vi "diagnostics.vi"(0 "Path Data":T1={"Path"=[], "Target Velocities"=[], "Robot Location"=[], "Relative Robot Angle (rad)"=0.0, "Curvature"=0.0, "Lookahead Point"=[3064.399009129367, 18229.833030071386], "Lookahead Index"=8.422809037111724, "Closest Point"=[], "Closest Point Index"=0, "Left Velocity"=0.0, "Right Velocity"=0.0, "Left Encoder Vel"=0, "Right Encoder Vel"=0, "Left Encoder Pos"=0, "Right Encoder Pos"=0, "Inital Robot Angle (deg)"=0.0}) -> (4 "Path":T4(graph)=[{"Smooth Path"=[0.0, 3.9831976339745525, 8.918786774310743, 15.996756278926227, 26.94310215462526, 44.45175679243214, 72.85576199340136, 119.21333672590853, 195.06952147459873, 319.3449114169336, 523.0654465520985, 857.1178508590853, 1404.971654642396, 2303.5684955547395, 3415.918100969553, 4658.468244850319, 5980.216850342943, 7349.961644912561, 8748.499353660785, 10163.825114581763, 11588.130666803412, 13015.85297046767, 14442.283167634836, 15862.389189218296, 17269.55815292861, 18653.942887255045, 20000.0], "Smooth Path"=[0.0, 2604.6593521886216, 5208.4834070465695, 7810.428161388078, 10408.979451847843, 13001.776283234469, 15585.016727668002, 18152.511956181766, 20694.135215630122, 23193.291890529486, 25622.77148689383, 27937.944042539046, 30065.60256829882, 32209.66168633789, 34363.622817575204, 36523.46279208931, 38686.62801955882, 40851.39631476969, 43016.44613594504, 45180.526806154805, 47342.144596973565, 49499.19086028001, 51648.41344856078, 53784.60445996854, 55899.29829439407, 57978.65493411005, 60000.0]}, {"Smooth Path"=[-155.34781165121697, -32.634161371312175], "Smooth Path"=[-10126.308473842537, -2127.2496942088364]}, {"Smooth Path"=[0.0], "Smooth Path"=[0.0]}, {"Smooth Path"=[0.0, -155.34781165121697], "Smooth Path"=[0.0, -10126.308473842537]}], 6 "Robot Angle (deg)":dbl=-0.87890625, 8 "Target Velocities":cluster{dbl, dbl}(graph)={850.0, 850.0}, 10 "Left Velocity":T2(graph)={"Quadrature Velocity"=0, "Left Velocity"=850.0}, 15 "Right Velocity":T3(graph)={"Quadrature Velocity"=0, "Right Velocity"=850.0})   [LabVIEW 2018]
uses:
  path data.ctl
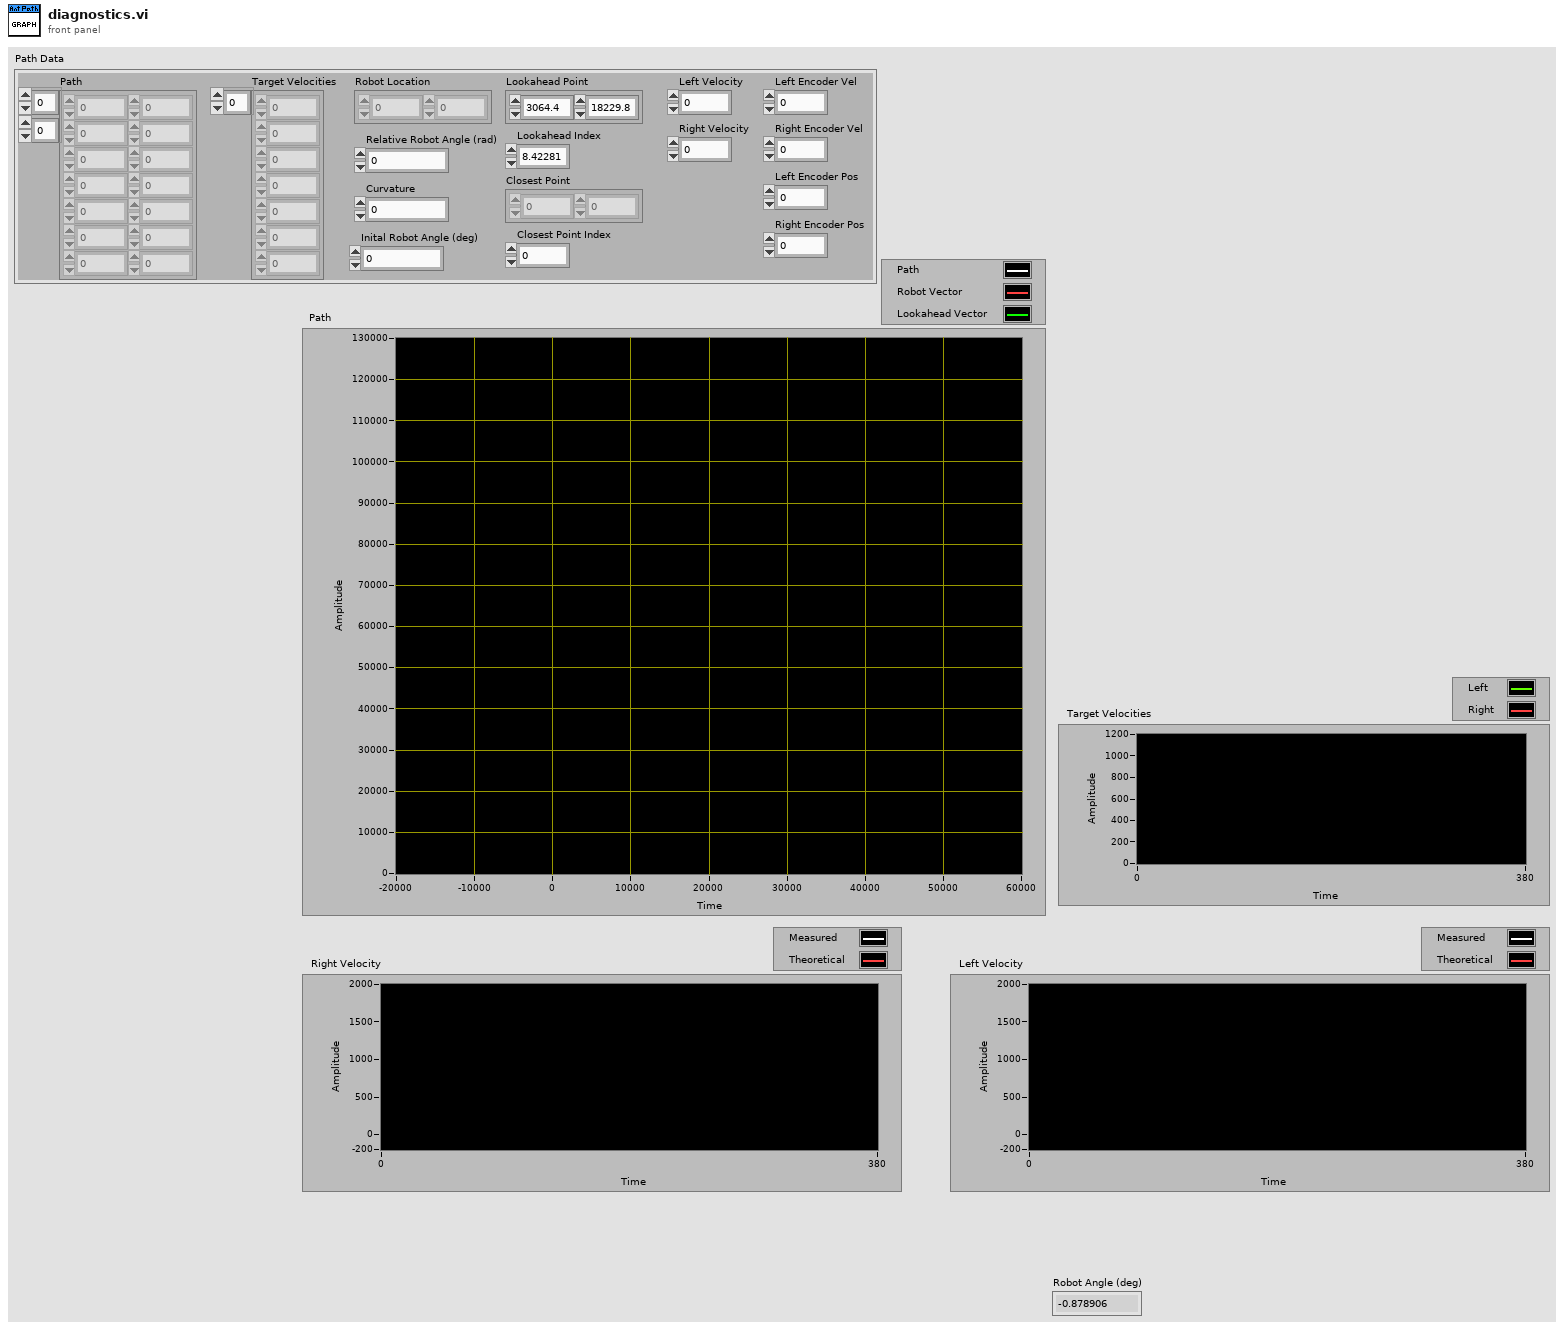
[diagram p1: front panel]
types:
  T1 = typedef "path data.ctl" = cluster{"Path":dbl[][], "Target Velocities":dbl[], "Robot Location":dbl[], "Relative Robot Angle (rad)":dbl, "Curvature":dbl, "Lookahead Point":dbl[], "Lookahead Index":dbl, "Closest Point":dbl[], "Closest Point Index":i32, "Left Velocity":dbl, "Right Velocity":dbl, "Left Encoder Vel":i32, "Right Encoder Vel":i32, "Left Encoder Pos":i32, "Right Encoder Pos":i32, "Inital Robot Angle (deg)":dbl}
  T2 = cluster{"Quadrature Velocity":i32, "Left Velocity":dbl}
  T3 = cluster{"Quadrature Velocity":i32, "Right Velocity":dbl}
  T4 = cluster{"Smooth Path":dbl[], "Smooth Path":dbl[]}[]
  T5 = cluster{"Left Velocity":dbl, "Right Velocity":dbl}
  T6 = cluster{"Left Encoder Vel":i32, "Left Velocity":dbl}
  T7 = cluster{"Right Encoder Vel":i32, "Right Velocity":dbl}
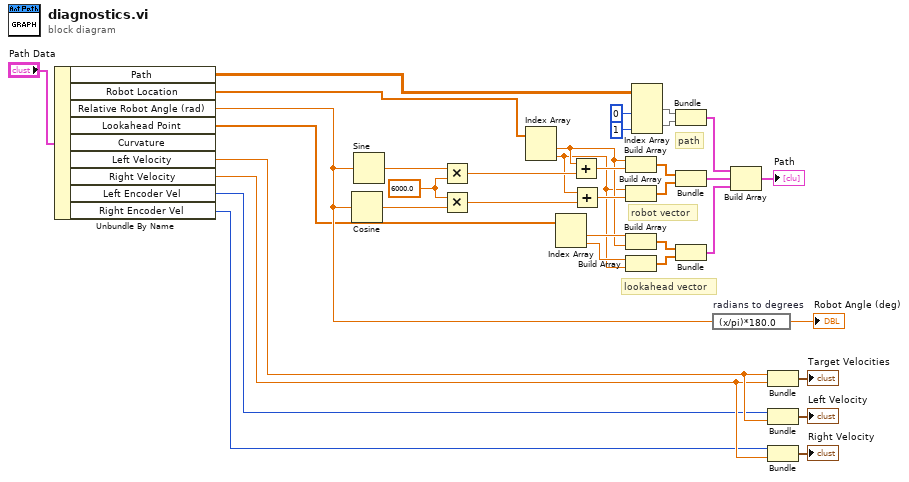
[diagram p0: block diagram]
diagram:
  w27 = 6000.0
  # "lookahead vector"
  # "robot vector"
  # "path"
  n1 = Unbundle By Name("Path Data") -> ("Path"=w8:dbl[][], "Robot Location"=w7:dbl[], "Relative Robot Angle (rad)"=w6:dbl, "Lookahead Point"=w5:dbl[], "Left Velocity"=w4:dbl, "Right Velocity"=w3:dbl, "Left Encoder Vel"=w2:i32, "Right Encoder Vel"=w1:i32)  [unwired: 1 out]
  n2 = Cosine(x=w6) -> (cos(x)=w28:dbl)
  n3 = Sine(x=w6) -> (sin(x)=w29:dbl)
  n4 = Multiply(x=w29, y=w27) -> (x*y=w26:dbl)
  n5 = Multiply(x=w27, y=w28) -> (x*y=w25:dbl)
  n6 = Index Array(array=w7) -> (element #1=w15:dbl, element #2=w14:dbl)  [unwired: 2 in]
  n7 = Index Array(array=w5) -> (element #1=w20:dbl, element #2=w18:dbl)  [unwired: 2 in]
  n8 = Add(x=w15, y=w26) -> (x+y=w24:dbl)
  n9 = Add(x=w14, y=w25) -> (x+y=w23:dbl)
  n10 = Build Array(w15, w24) -> (w33:dbl[])
  n11 = Build Array(w14, w23) -> (w32:dbl[])
  n12 = Build Array(w20, w15) -> (w22:dbl[])
  n13 = Build Array(w18, w14) -> (w21:dbl[])
  n14 = Index Array(array=w8, index (col) #1=0 ("disabled index (col)"), index (col) #2=1 ("index (col)")) -> (element #1=w36:dbl[], element #2=w16:dbl[])  [unwired: 2 in]
  n15 = Bundle("Path"=w36, "Path"=w16) -> (w17:cluster{"Path":dbl[], "Path":dbl[]})  [unwired: 1 in]
  n16 = Bundle(w33, w32) -> (w31:cluster{dbl[], dbl[]})  [unwired: 1 in]
  n17 = Bundle(w22, w21) -> (w19:cluster{dbl[], dbl[]})  [unwired: 1 in]
  n18 = expression code="(x/pi)*180.0" "radians to degrees"(w6) -> (→"Robot Angle (deg)":dbl)
  n19 = Build Array(w17, w31, w19) -> (→"Path":cluster{"Path":dbl[], "Path":dbl[]}[])
  n20 = Bundle("Left Velocity"=w4, "Right Velocity"=w3) -> (→"Target Velocities":T5)  [unwired: 1 in]
  n21 = Bundle("Left Encoder Vel"=w2, "Left Velocity"=w4) -> (→"Left Velocity":T6)  [unwired: 1 in]
  n22 = Bundle("Right Encoder Vel"=w1, "Right Velocity"=w3) -> (→"Right Velocity":T7)  [unwired: 1 in]
